vi "LuaVIEW CIN Wrapper.vi"(0 "action":T1, 1 "refnum in":refnum<vi>, 5 "LuaVIEW reference in":T2) -> (6 "LuaVIEW reference out":T2)   [LabVIEW 2013]
doc: "This is a non-reentrant wrapper around the reentrant CIN VI. This VI serves to improve memory usage and instantiation performance by reducing the number of reentrant data spaces. By calling infrequently used CIN actions that are not at risk of being contended through this VI instead of through the reentrant VI, a reentrant dataspace instantiation is saved with minimal impact on run-time performance. These dataspaces can amount to significant overhead because of the multiplier effect caused by templates and reentrant VIs containing calls to the reentrant CIN VI."
uses:
  typedefs/et_LuaVIEW CIN Actions.ctl
  typedefs/t_LuaVIEW Reference.ctl
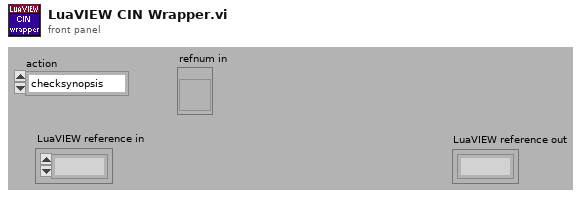
[diagram p1: front panel]
types:
  T1 = typedef "et_LuaVIEW CIN Actions.ctl" = enum16{"checksynopsis", "_open", "_registerpublic", "_registerexport", "__never_an_error_result_ns", "luaversion", "cinversion", "_totals", "_taskcount", "pathological", "_unregnextpublic", "registryusecount", "__per_state_actions", "regsetprivate", "regsetindex", "regsetmodule", "_revokeexports", "_usepublic", "prepare", "compile", "execute", "call", "unregstaterefs", "_close", "pullboolean", "pullnumber", "pullI8", "pullU8", "pullI16", "pullU16", "pullI32", "pullU32", "pullobject", "pullrefnum", "pullstring", "pullflat", "pushflat", "pushobject", "getattribute", "setattribute", "stacktostring", "_startyieldtest", "_endyieldtest", "_pollprintbuffer", "__never_an_error_result_ps", "_pollexport", "setclone", "forcecleanup", "gettop", "clearstack", "insert", "pushboolean", "pushnumber", "pushrefnum", "pushstring", "pushnil", "pushvalue", "gettaskref", "settaskref"}
  T2 = typedef "t_LuaVIEW Reference.ctl" = refnum<k1>
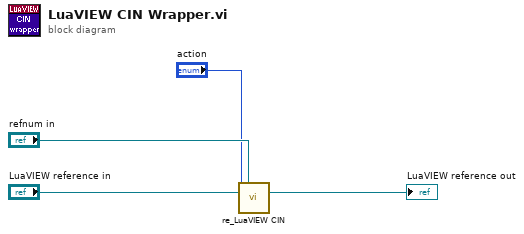
[diagram p0: block diagram]
diagram:
  n1 = call "re_LuaVIEW CIN.vi"("action"="action", "refnum in"="refnum in", "LuaVIEW reference in"="LuaVIEW reference in") -> ("LuaVIEW reference out"=→"LuaVIEW reference out":T2)  [unwired: 6 in, 6 out]
